vi "多影像平均_二值化_抓邊.vi"() -> ()   [LabVIEW 2015]
uses:
  <vilib>/vision/Measure.llb/Edge Options.ctl
  <vilib>/vision/Measure.llb/Edge Polarity.ctl
  <vilib>/userdefined/High Color/IMAQdx.ctl
  <vilib>/Utility/miscctls.llb/LVPositionTypeDef.ctl
  <vilib>/vision/NI_Vision_Development_Module.lvlib
  <vilib>/vision/driver/NI_Vision_Acquisition_Software.lvlib
  <resource>/objmgr/imaqdx.rc
panel:
  in  "Rectangle 2":T1={"Left"=208, "Top"=416, "Right"=273, "Bottom"=496, "Rotation"=0.0} {"Rotation" format="%.2f"; "Left" scale=0.0..1024.0; "Right" scale=0.0..1024.0}
  in  "載入影像":bool
  in  "拍攝影像":bool
  in  "影像數量":i32=4
  out "二值化影像陣列":T2[](array[plugin-control])
  out "全部影像Histograph":T3(graph)
  out "Image binary":T2(plugin-control)
  out "平均影像Histograph":T4(graph)
  out "Standard Deviation":sgl format="%#.2f"
  out "Mean":sgl format="%#.2f"
  out "影像陣列":T2[](array[plugin-control])
  in  "stop":bool
  in  "Horizontal Progress Bar":u8(slide) scale=0.0..255.0
  out "Image mean":T2(plugin-control)
  out "取像編號":i32
  out "取像視窗":T2(plugin-control)
  in  "Session In":T5="cam1"
  out "degrees":sgl
  in  "單點":bool
  in  "Edge Options":T6={"Edge Polarity"=0, "Kernel Size"=3, "Width"=3, "Minimum Edge Strength"=10.0, "Interpolation Type"=enum."Bilinear Fixed", "Data Processing Method"=enum."Average"} {"Edge Polarity" items=["All Edges", "Rising Edges", "Falling Edges"]; "Minimum Edge Strength" format="%.2f"; "Width" step=2; "Kernel Size" step=2}
  out "Gradient Information":dbl[][](graph)
  out "Line Segment":T8 {"Point 2"."Y" format="%.2f"; "Point 2"."X" format="%.2f"; "Point 1"."Y" format="%.2f"; "Point 1"."X" format="%.2f"}
  out "error out":errorcluster
  in  "Direction":T9(ring)
  in  "Process":u16(ring) items=["Get First Edge", "Get First + Last Edge", "Get All Edges", "Get Best Edge"]
  out "Line Profile":T10(graph)
  in  "Gap":i32=10 min=1 max=300
  out "Image":T2(plugin-control)
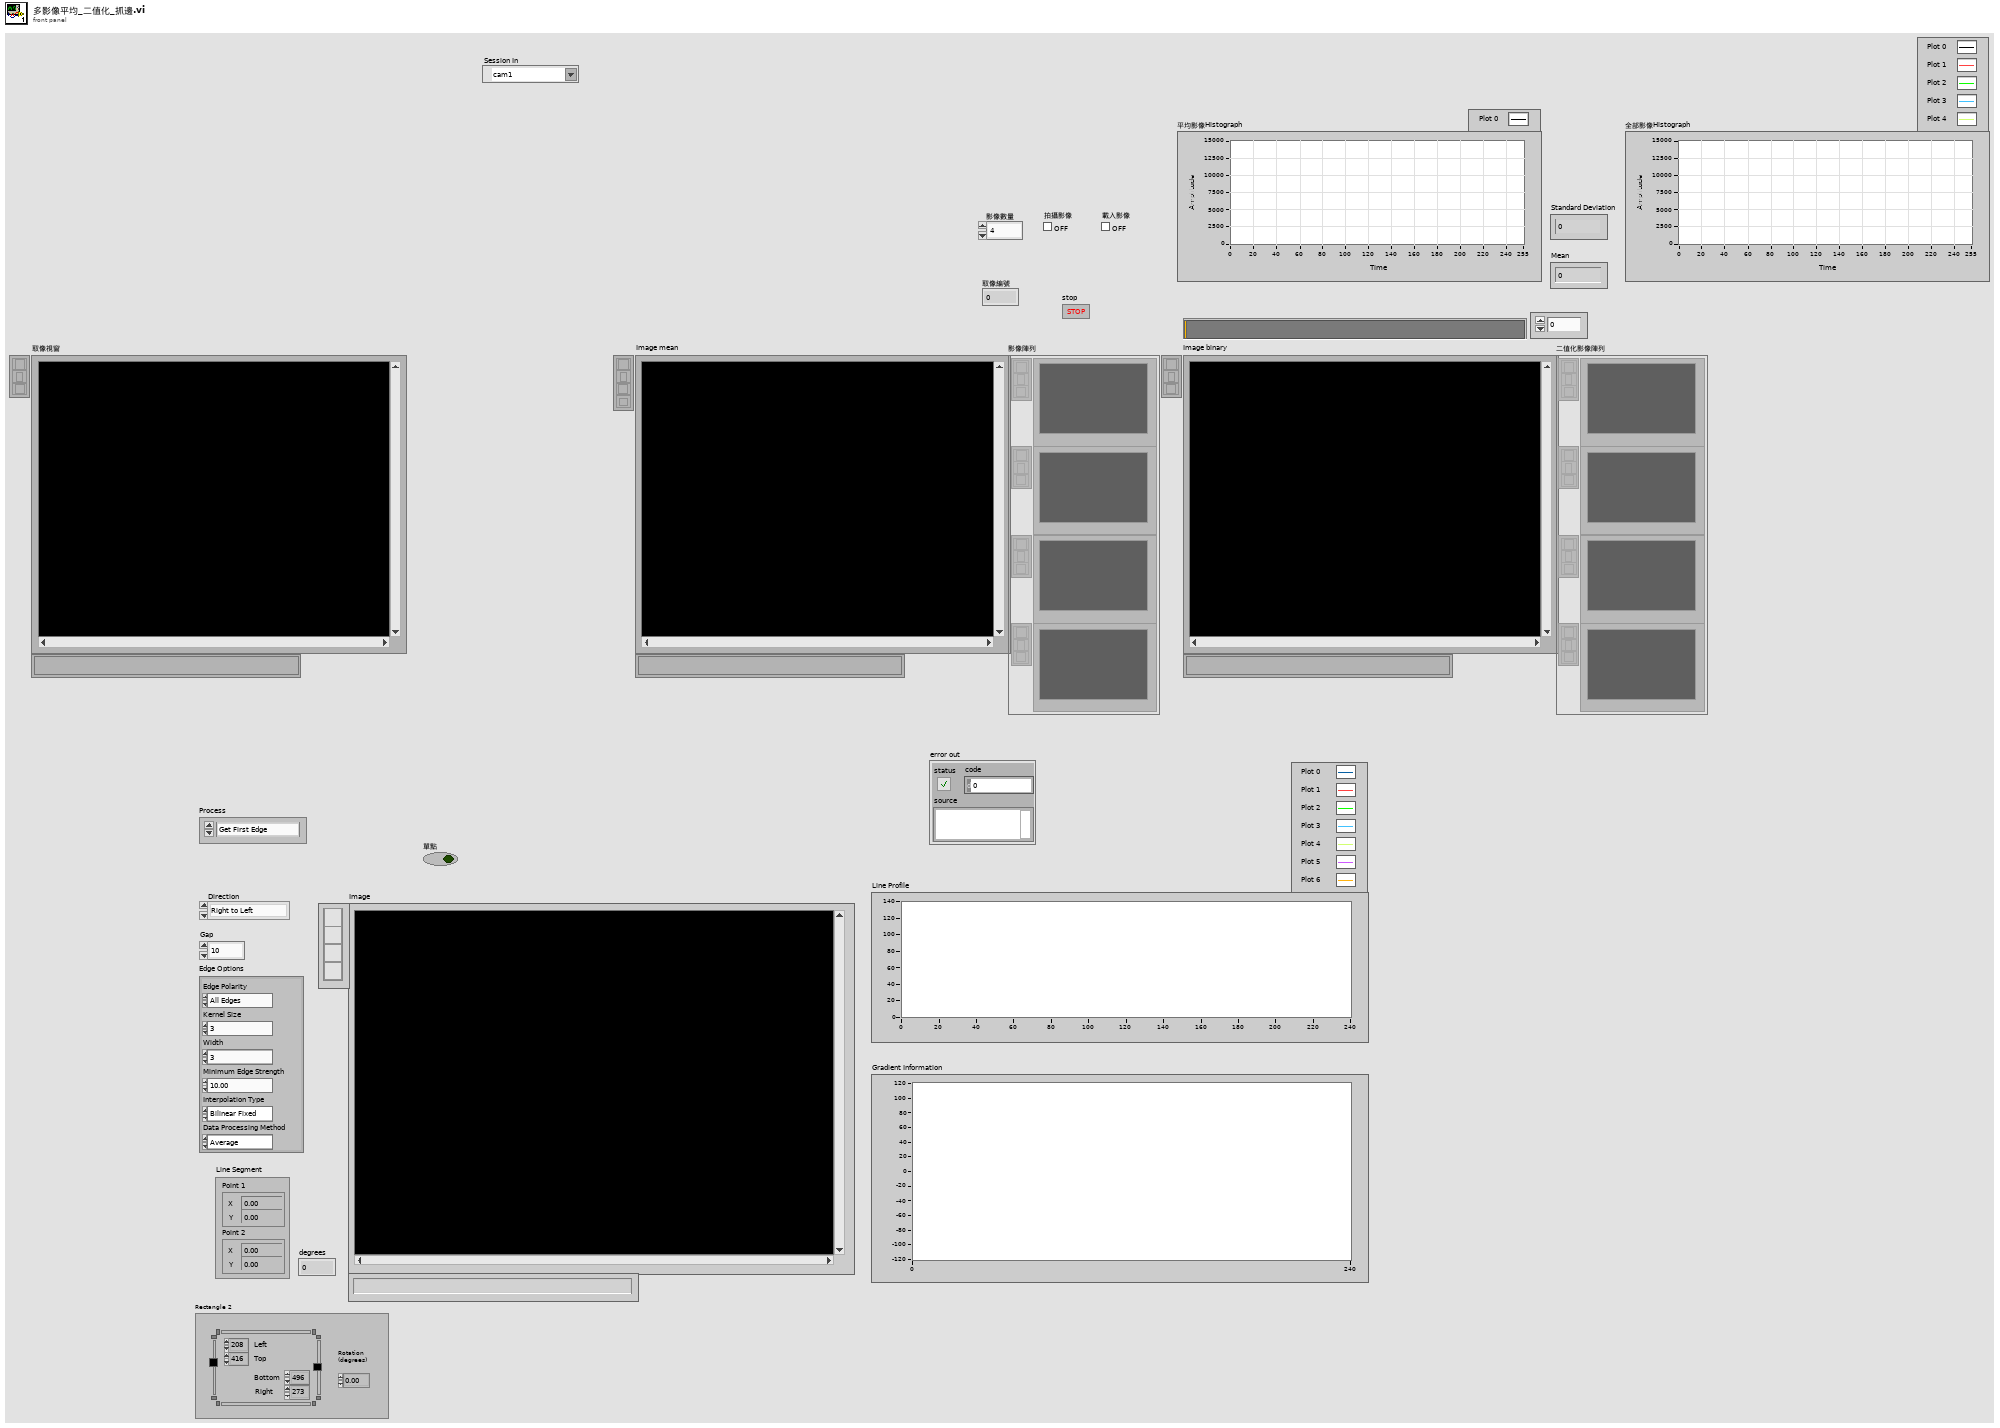
[diagram p1: front panel]
types:
  T1 = typedef "IMAQ Rectangle" = cluster{"Left":i32, "Top":i32, "Right":i32, "Bottom":i32, "Rotation":dbl}
  T2 = typedef "IMAQ Image.ctl" = refnum<image>
  T3 = cluster{"Starting Value":sgl, "Incremental Value":sgl, "Histogram":u32[]}[]
  T4 = cluster{"Starting Value":sgl, "Incremental Value":sgl, "Histogram":u32[]}
  T5 = typedef "IMAQdx.ctl" = refnum<k21>
  T6 = typedef "Edge Options.ctl" = cluster{"Edge Polarity":T7, "Kernel Size":u32, "Width":u32, "Minimum Edge Strength":sgl, "Interpolation Type":enum32{"Zero Order", "Bilinear", "Quadratic", "Cubic", "Bilinear Fixed"}, "Data Processing Method":enum32{"Average", "Median"}}
  T7 = typedef "Edge Polarity.ctl" = u32
  T8 = cluster{"Point 1":cluster{"X":sgl, "Y":sgl}, "Point 2":cluster{"X":sgl, "Y":sgl}}
  T9 = enum16{"Right to Left", "Left  to Right", "Up to Down", "Down to Up"}
  T10 = cluster{"x0":sgl, "dx":sgl, "Pixels Line":sgl[]}[]
  T11 = typedef "LVPositionTypeDef.ctl" = cluster{"Left":i32, "Top":i32}
  T12 = typedef "Image Type" = u32
  T13 = cluster{"Global Rectangle":i32[], "Contours":cluster{"Contour Type":u32, "ROI Type":u32, "Points":i32[]}[]}
  T14 = typedef "IMAQ Line" = cluster{"Start X":i32, "Start Y":i32, "End X":i32, "End Y":i32}
  T15 = cluster{"Point 1":cluster{"x":dbl, "y":dbl}, "Point 2":cluster{"x":dbl, "y":dbl}}
  T16 = typedef "ROI Descriptor" = cluster{"Global Rectangle":i32[], "Contours":cluster{"ID":enum32{"External", "Internal"}, "Type":u32, "Coordinates":i32[]}[]}
  T17 = typedef "IMAQ Point" = cluster{"X":sgl, "Y":sgl}
  T18 = typedef "Edge New.ctl" = cluster{"Location (Pixel)":cluster{"X":sgl, "Y":sgl}, "Location (Real-World)":cluster{"X":sgl, "Y":sgl}, "Distance (Pixel)":dbl, "Distance (Real-World)":dbl, "Strength":dbl, "Noise":dbl, "Rising?":bool}
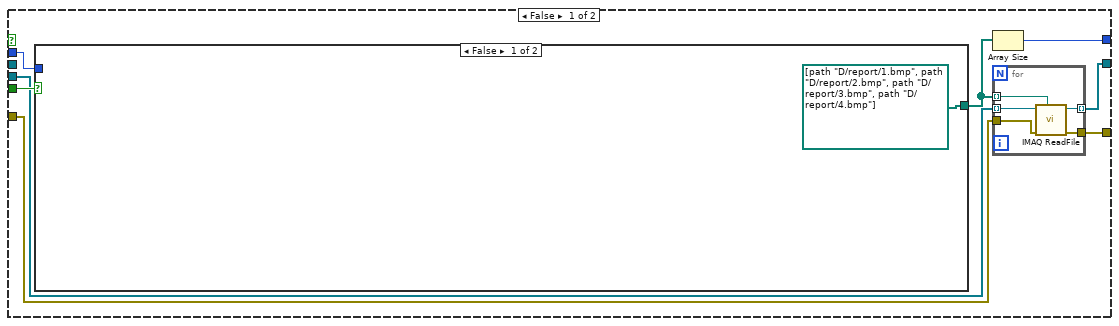
[diagram p2: hidden frame]
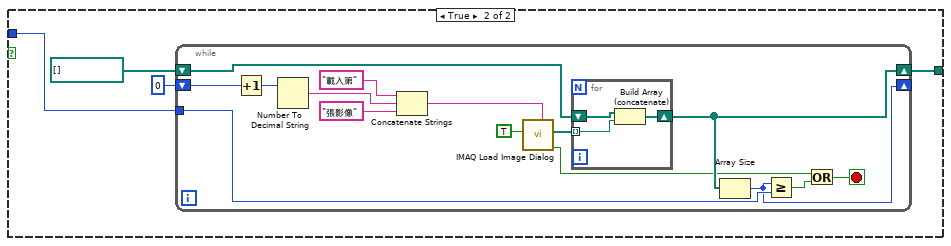
[diagram p3: hidden frame]
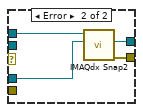
[diagram p4: hidden frame]
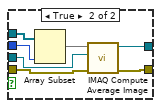
[diagram p5: hidden frame]
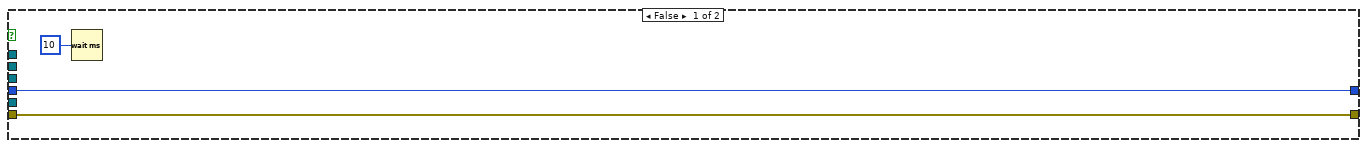
[diagram p6: hidden frame]
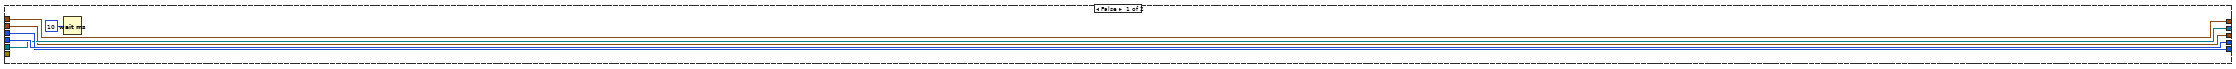
[diagram p8: hidden frame]
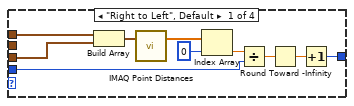
[diagram p9: hidden frame]
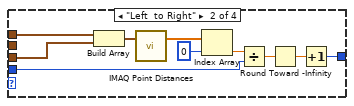
[diagram p10: hidden frame]
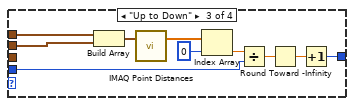
[diagram p11: hidden frame]
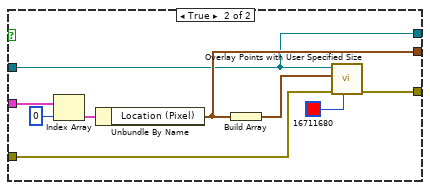
[diagram p14: hidden frame]
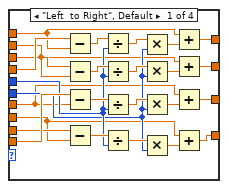
[diagram p15: hidden frame]
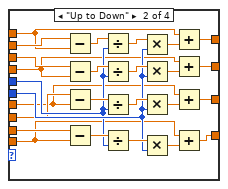
[diagram p16: hidden frame]
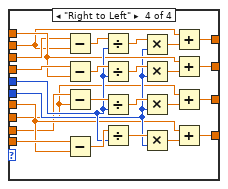
[diagram p17: hidden frame]
diagram:
  w40 = T12 0 items=["Grayscale (U8)", "Grayscale (I16)", "Grayscale (SGL)", "Complex (CSG)", "RGB (U32)", "HSL (U32)", "RGB (U64)", "Grayscale (U16)"] ("Image Type")
  w42 = i32[] [2] items=["No  event", "Click event", "Draw event", "Move event", "Size event", "Scroll event", "Activate event", "Close event", "Double click event"] ("Events list (all)")
  n1 = property on="Image" class="ImageControl"("ROI"=T13 {"Global Rectangle"=[450, 180, 600, 400], "Contours"=[{"Contour Type"=0, "ROI Type"=3, "Points"=[450, 180, 600, 400]}]}) -> ()  [unwired: 2 in, 2 out]
  n2 = property on="Pane" class="Pane"("Origin"=T11 {"Left"=-5267, "Top"=-1496} ("Position")) -> (error out=w5:errorcluster)  [unwired: 2 in, 1 out]
  n3 = flat-sequence {
    tunnel: [w68] -> w38
    tunnel: [w67] -> w37
    tunnel: [w65] -> w36
    tunnel: "影像數量" -> [w61]
    tunnel: [w63] -> w35
    tunnel: "拍攝影像" -> [w63]
    tunnel: [w62] -> w34
    tunnel: "載入影像" -> [w62]
    tunnel: [w61] -> w33
    tunnel: [w60] -> w32
    tunnel: [w57] -> w31
    tunnel: [w55] -> w30
    tunnel: [w53] -> w29
    tunnel: [w46] -> w28
    tunnel: w5 -> [w45]
    tunnel: w38 -> [w103]
    tunnel: w37 -> [w104]
    tunnel: [w102] -> w27
    tunnel: w36 -> [w101]
    tunnel: [w101] -> w26
    tunnel: w35 -> [w100]
    tunnel: w34 -> [w99]
    tunnel: w33 -> [w98]
    tunnel: [w97] -> w25
    tunnel: [w96] -> w24
    tunnel: w32 -> [w95]
    tunnel: [w95] -> w23
    tunnel: [w94] -> w22
    tunnel: w31 -> [w94]
    tunnel: w30 -> [w93]
    tunnel: [w93] -> w21
    tunnel: [w92] -> w20
    tunnel: w29 -> [w92]
    tunnel: w28 -> [w91]
    tunnel: w27 -> [w177]
    tunnel: w26 -> [w182]
    tunnel: w25 -> [w181]
    tunnel: w24 -> [w174]
    tunnel: w23 -> [w180]
    tunnel: [w180] -> w19
    tunnel: [w171] -> w18
    tunnel: [w177] -> w17
    tunnel: [w176] -> w16
    tunnel: [w179] -> w15
    tunnel: w22 -> [w179]
    tunnel: w21 -> [w175]
    tunnel: [w175] -> w14
    tunnel: [w178] -> w13
    tunnel: w20 -> [w178]
    tunnel: w19 -> [w202]
    tunnel: w18 -> [w197]
    tunnel: w17 -> [w203]
    tunnel: w16 -> [w195]
    tunnel: w15 -> [w201]
    tunnel: w14 -> [w196]
    tunnel: w13 -> [w198]
    tunnel: [w195] -> w9
    tunnel: [w194] -> w4
    frame #0 {
      w59 = T12 0 items=["Grayscale (U8)", "Grayscale (I16)", "Grayscale (SGL)", "Complex (CSG)", "RGB (U32)", "HSL (U32)", "RGB (U64)", "Grayscale (U16)"] ("Image Type")
      w52 = 20
      w64 = T12 0 items=["Grayscale (U8)", "Grayscale (I16)", "Grayscale (SGL)", "Complex (CSG)", "RGB (U32)", "HSL (U32)", "RGB (U64)", "Grayscale (U16)"] ("Image Type")
      n4 = call <vilib>:"IMAQdx Open Camera.vi"("error in"=w45, "Session In"="Session In") -> ("error out"=w54:errorcluster, "Session Out"=w68:T5)  [unwired: 8 in]
      n5 = for {
        N: w52 -> [_]
        tunnel: [w90] -> w67 mode=indexing
        tunnel: w54 -> [w89]
        tunnel: [w88] -> w51
        i -> [w87]
        n6 = Number To Decimal String(number=w87) -> (decimal integer string=w85:string)  [unwired: 1 in]
        n7 = Concatenate Strings("Image", w85) -> (w84:string)
        n8 = call "IMAQ Create"("Image Name"=w84, "error in (no error)"=w89) -> ("New Image"=w90:T2, "error out"=w88:errorcluster)  [unwired: 3 in]
      }
      n9 = for {
        N: w52 -> [_]
        tunnel: [w76] -> w53 mode=indexing
        tunnel: w51 -> [w75]
        tunnel: [w70] -> _
        tunnel: [w70] -> w50 mode=indexing
        i -> [w74]
        n10 = Number To Decimal String(number=w74) -> (decimal integer string=w72:string)  [unwired: 1 in]
        n11 = Concatenate Strings("Histogram Mask", w72) -> (w71:string)
        n12 = call "IMAQ Create"("Image Name"=w71, "error in (no error)"=w75) -> ("New Image"=w76:T2, "error out"=w70:errorcluster)  [unwired: 3 in]
      }
      n13 = for {
        N: w52 -> [_]
        tunnel: [w83] -> w60 mode=indexing
        tunnel: w50 -> [w82] mode=indexing
        tunnel: [w81] -> w47
        i -> [w80]
        n14 = Number To Decimal String(number=w80) -> (decimal integer string=w78:string)  [unwired: 1 in]
        n15 = Concatenate Strings("Threshole", w78) -> (w77:string)
        n16 = call "IMAQ Create"("Image Name"=w77, "error in (no error)"=w82) -> ("New Image"=w83:T2, "error out"=w81:errorcluster)  [unwired: 3 in]
      }
      n17 = call "IMAQ Create"("Image Name"="imageMeans", "Image Type"=w64, "error in (no error)"=w47) -> ("New Image"=w65:T2, "error out"=w49:errorcluster)  [unwired: 2 in]
      n18 = call "IMAQ Create"("Image Name"="Histogram Mask", "error in (no error)"=w49) -> ("New Image"=w55:T2, "error out"=w48:errorcluster)  [unwired: 3 in]
      n19 = call "IMAQ Create"("Image Name"="imageBinary", "Image Type"=w59, "error in (no error)"=w48) -> ("New Image"=w57:T2, "error out"=w46:errorcluster)  [unwired: 2 in]
    }
    frame #1 {
      n20 = case shown="True" w100 {
        tunnel: w104 -> [w109 w148]
        tunnel: w103 -> [_ w147]
        tunnel: w91 -> [w108 w145]
        tunnel: [w110 w144] -> w102
        tunnel: w99 -> [w112 _]
        tunnel: w98 -> [w111 w142]
        tunnel: [w107 w143] -> w97
        tunnel: [w105 w142] -> w96
        frame False {
          n21 = case shown="False" w112 {
            tunnel: [path[] [path "D:/report/1.bmp", path "D:/report/2.bmp", path "D:/report/3.bmp", path "D:/report/4.bmp"] w117] -> w106
            tunnel: w111 -> [_ w116]
            frame False {
            }
            frame True {
              n22 = while {
                tunnel: w116 -> [w129]
                shift-right: [w132] -> w117
                shift-left: path[] [] -> [w128]
                shift-right: [w127] -> _
                shift-left: 0 -> [w126]
                stop <- w119 stop-if-true
                n23 = Increment(x=w126) -> (x+1=w125:i32)
                n24 = Number To Decimal String(number=w125) -> (decimal integer string=w122:string)  [unwired: 1 in]
                n25 = Concatenate Strings("載入第", w122, "張影像") -> (w121:string)
                n26 = call "IMAQ Load Image Dialog"("Button Label"=w121, "Multiple Files? (No)"=TRUE) -> ("Cancelled?"=w120:bool, "Paths"=w130:path[])  [unwired: 7 in, 1 out]
                n27 = for {
                  tunnel: w130 -> [w134] mode=indexing
                  shift-right: [w133] -> w132
                  shift-left: w128 -> [w135]
                  n28 = Build Array (concatenate)(w135, w134) -> (w133:path[])
                }
                n29 = Array Size(array=w132) -> (size(s)=w127:i32)
                n30 = Greater Or Equal?(x=w127, y=w129) -> (x >= y?=w118:bool)
                n31 = Or(x=w120, y=w118) -> (x .or. y?=w119:bool)
              }
            }
          }
          n32 = Array Size(array=w106) -> (size(s)=w105:i32)
          n33 = for {
            tunnel: w106 -> [w140] mode=indexing
            tunnel: [w139] -> w110 mode=indexing
            tunnel: w109 -> [w138] mode=indexing
            tunnel: w108 -> [w137]
            tunnel: [w136] -> w107
            n34 = call "IMAQ ReadFile"("File Path"=w140, "error in (no error)"=w137, "Image"=w138) -> ("error out"=w136:errorcluster, "Image Out"=w139:T2)  [unwired: 4 in, 3 out]
          }
        }
        frame True {
          n35 = for {
            N: w142 -> [_]
            tunnel: w148 -> [w151] mode=indexing
            tunnel: w147 -> [w149]
            tunnel: dbl[] [0.01, 0.03, 0.05, 0.07] -> [w159] mode=indexing
            tunnel: w145 -> [w154]
            tunnel: [w158] -> w144 mode=indexing
            tunnel: [w156] -> w143
            i -> [w160]
            w157 = T12 0 items=["Grayscale (U8)", "Grayscale (I16)", "Grayscale (SGL)", "Complex (CSG)", "RGB (U32)", "HSL (U32)", "RGB (U64)", "Grayscale (U16)"] ("Image Type")
            n36 = property class="IMAQdx"(reference=w149, error in=w154, "ActiveAttribute"="CameraAttributes::Exposure::Value", "ValueDBL"=w159) -> (reference out=w150:T5, error out=w152:errorcluster)
            n37 = case shown="No Error" w152 {
              tunnel: [w165 w169] -> w156
              tunnel: [w164 w166] -> w155
              tunnel: w152 -> [w163 _]
              tunnel: w150 -> [w162 _]
              tunnel: w151 -> [w161 w168]
              tunnel: w149 -> [_ w167]
              frame No Error {
                n38 = call <vilib>:"IMAQdx Snap2.vi"("error in"=w163, "Image In"=w161, "Session In"=w162) -> ("error out"=w165:errorcluster, "Image Out"=w164:T2)  [unwired: 6 in, 1 out]
              }
              frame Error {
                n39 = call <vilib>:"IMAQdx Snap2.vi"("Image In"=w168, "Session In"=w167) -> ("error out"=w169:errorcluster, "Image Out"=w166:T2)  [unwired: 7 in, 1 out]
              }
            }
            "取像視窗" <- w155
            n40 = call "IMAQ Cast Image"("Image Type"=w157, "Image Src"=w155) -> ("Image Dst Out"=w158:T2)  [unwired: 8 in, 1 out]
            "取像編號" <- w160
          }
          n41 = property on="Pane" class="Pane"("Origin"=T11 {"Left"=-6573, "Top"=-1496} ("Position")) -> ()  [unwired: 2 in, 2 out]
        }
      }
    }
    frame #2 {
      n42 = Not Equal?(x=w174, y=1) -> (x != y?=w172:bool)
      n43 = case shown="False" w172 {
        tunnel: w182 -> [_ w193]
        tunnel: w181 -> [w186 w192]
        tunnel: w174 -> [_ w191]
        tunnel: [w186 w189] -> w171
        tunnel: w177 -> [w184 w188]
        tunnel: [w183 w187] -> w176
        frame False {
          n44 = Index Array(array=w184, index=0) -> (element=w183:T2)
        }
        frame True {
          n45 = Array Subset(array=w188, length=w191) -> (w190:T2[])  [unwired: 1 in]
          n46 = call "IMAQ Compute Average Image"("error in (no error)"=w192, "Image Dst"=w193, "Images"=w190) -> ("error out"=w189:errorcluster, "Image Dst Out"=w187:T2)  [unwired: 7 in]
        }
      }
      "Image mean" <- w176
      n47 = property on="Pane" class="Pane"("Origin"=T11 {"Left"=-5267, "Top"=-1496} ("Position")) -> ()  [unwired: 2 in, 2 out]
    }
    frame #3 {
      w199 = i32[] [2] items=["No  event", "Click event", "Draw event", "Move event", "Size event", "Scroll event", "Activate event", "Close event", "Double click event"] ("Events list (all)")
      n48 = property on="Image mean" class="ImageControl"("ROI"=T13 {"Global Rectangle"=[0, 0, 1292, 964], "Contours"=[{"Contour Type"=0, "ROI Type"=3, "Points"=[0, 0, 1292, 964]}]}) -> ()  [unwired: 2 in, 2 out]
      n49 = while {
        tunnel: w203 -> [w223]
        tunnel: w202 -> [w222]
        tunnel: w195 -> [w220]
        tunnel: w196 -> [w221]
        tunnel: w201 -> [w219]
        tunnel: w199 -> [w217]
        shift-right: [w214] -> _
        shift-left: _ -> [w212]
        tunnel: w198 -> [w207]
        tunnel: w197 -> [w206]
        tunnel: [w204] -> w194
        i -> [w215]
        stop <- "stop" stop-if-true
        n50 = invoke on="Image mean" class="ImageControl" method="Get Last Event"("Which Events"=w217) -> ("Type"=w216:i32)  [unwired: 7 in, 7 out]
        n51 = property on="平均影像Histograph" class="WFGraph (strict)"() -> ("YScale.Maximum"=w205:dbl)  [unwired: 2 in, 2 out]
        n52 = property on="全部影像Histograph" class="WFGraph (strict)"("YScale.Maximum"=w205) -> ()  [unwired: 2 in, 2 out]
        n53 = Not Equal?(x="Horizontal Progress Bar", y=w212) -> (x != y?=w209:bool)
        n54 = Not Equal To 0?(x=w216) -> (x != 0?=w210:bool)
        n55 = Equal To 0?(x=w215) -> (x = 0?=w211:bool)
        n56 = Compound Arithmetic op=OR(w211, w210, w209) -> (w208:bool)
        n57 = case shown="True" w208 {
          tunnel: w223 -> [_ w232]
          tunnel: w222 -> [_ w260]
          tunnel: w221 -> [_ w229]
          tunnel: w220 -> [_ w230]
          tunnel: w219 -> [_ w247]
          tunnel: "Horizontal Progress Bar" -> [w225 w245]
          tunnel: [w225 w245] -> w214
          tunnel: w207 -> [_ w243]
          tunnel: w206 -> [w224 w234]
          tunnel: [w224 w227] -> w204
          frame False {
            n58 = Wait (ms)(milliseconds to wait=u32 10) -> ()  [unwired: 1 out]
          }
          frame True {
            n59 = property on="Image mean" class="ImageControl"() -> ("ROI"=w242:T13)  [unwired: 2 in, 2 out]
            n60 = property on="Image binary" class="ImageControl"("Zoom to Fit Mode"=TRUE) -> ()  [unwired: 2 in, 2 out]
            n61 = call "IMAQ Convert ROI to Rectangle"("error in (no error)"=w234, "ROI Descriptor"=w242) -> ("error out"=w235:errorcluster, "Rectangle"=w252:T1)  [unwired: 7 in]
            n62 = Unbundle By Name(w252) -> ("Left"=w248:i32, "Top"=w249:i32, "Right"=w250:i32, "Bottom"=w251:i32)
            n63 = Build Array(w248, w249, w250, w251) -> (w241:i32[])
            n64 = for {
              tunnel: w232 -> [w263] mode=indexing
              tunnel: w260 -> [w277] mode=indexing
              tunnel: [w276] -> w259 mode=indexing
              tunnel: [w264] -> w255 mode=indexing
              tunnel: w245 -> [w273]
              tunnel: w243 -> [w270] mode=indexing
              tunnel: w242 -> [w272]
              tunnel: w241 -> [w271]
              tunnel: [w267] -> w236
              tunnel: w235 -> [w266]
              tunnel: [w265] -> w231 mode=indexing
              n65 = call "IMAQ ROIToMask"("error in (no error)"=w266, "ROI Descriptor"=w272, "Image"=w270, "Image Model"=w263) -> ("error out"=w269:errorcluster, "Image Out"=w262:T2)  [unwired: 2 in, 1 out]
              n66 = call "IMAQ Extract 2"("Optional Rectangle"=w271, "error in (no error)"=w269, "Image Dst"=w270, "Image Src"=w263) -> ("error out"=w268:errorcluster, "Image Dst Out"=w265:T2)  [unwired: 6 in]
              n67 = Bundle By Name(cluster=cluster{"Lower value":sgl, "Upper value":sgl} {"Lower value"=128.0, "Upper value"=255.0} ("Range"), "Lower value"=w273) -> (w274:cluster{"Lower value":sgl, "Upper value":sgl})
              n68 = call "IMAQ Histograph"("error in (no error)"=w268, "Image"=w262) -> ("error out"=w261:errorcluster, "Histogram Graph"=w264:T4)  [unwired: 6 in, 2 out]
              n69 = call "IMAQ Threshold"("error in (no error)"=w261, "Range"=w274, "Image Dst"=w277, "Image Src"=w265) -> ("error out"=w267:errorcluster, "Image Dst Out"=w276:T2)  [unwired: 6 in]
            }
            "二值化影像陣列" <- w259
            "影像陣列" <- w231
            n70 = call "IMAQ ROIToMask"("error in (no error)"=w236, "ROI Descriptor"=w242, "Image"=w229, "Image Model"=w230) -> ("error out"=w239:errorcluster, "Image Out"=w228:T2)  [unwired: 2 in, 1 out]
            n71 = call "IMAQ Extract 2"("Optional Rectangle"=w241, "error in (no error)"=w239, "Image Dst"=w229, "Image Src"=w230) -> ("error out"=w238:errorcluster, "Image Dst Out"=w240:T2)  [unwired: 6 in]
            n72 = call "IMAQ Histograph"("error in (no error)"=w238, "Image"=w228) -> ("error out"=w237:errorcluster, "Standard  Deviation"=→"Standard Deviation":sgl, "Mean Value"=→"Mean":sgl, "Histogram Graph"=w253:T4)  [unwired: 6 in]
            "平均影像Histograph" <- w253
            n73 = Bundle By Name(cluster=cluster{"Lower value":sgl, "Upper value":sgl} {"Lower value"=128.0, "Upper value"=255.0} ("Range"), "Lower value"=w245) -> (w258:cluster{"Lower value":sgl, "Upper value":sgl})
            n74 = Build Array (concatenate)(w253, w255) -> (→"全部影像Histograph":T3)
            n75 = call "IMAQ Threshold"("error in (no error)"=w237, "Range"=w258, "Image Dst"=w247, "Image Src"=w240) -> ("error out"=w227:errorcluster, "Image Dst Out"=→"Image binary":T2)  [unwired: 6 in]
          }
        }
      }
    }
  }
  n76 = property on="Pane" class="Pane"(error in=w4, "Origin"=T11 {"Left"=-5844, "Top"=-513} ("Position")) -> (error out=w3:errorcluster)  [unwired: 1 in, 1 out]
  n77 = call "IMAQ Create"("Image Name"="Edge Detection Source", "error in (no error)"=w3) -> ("New Image"=w7:T2, "error out"=w6:errorcluster)  [unwired: 3 in]
  n78 = call "IMAQ Copy"("Image Dst"=w7, "Image Src"=w9) -> ("Image Dst Out"=w8:T2)  [unwired: 4 in, 1 out]
  n79 = call "IMAQ Cast Image"("Image Type"=w40, "error in (no error)"=w6, "Image Src"=w8) -> ("error out"=w39:errorcluster, "Image Dst Out"=w41:T2)  [unwired: 7 in]
  n80 = while {
    tunnel: w39 -> [w299]
    tunnel: w41 -> [w300]
    tunnel: w42 -> [w282]
    shift-right: [w297] -> _
    shift-left: _ -> [w296]
    shift-right: [w289] -> _
    shift-left: _ -> [w290]
    shift-right: [w284] -> _
    shift-left: _ -> [w285]
    shift-right: [w281] -> _
    shift-left: _ -> [w280]
    stop <- FALSE stop-if-true
    n81 = invoke on="Image" class="ImageControl" method="Get Last Event"("Which Events"=w282) -> ("Type"=w298:i32)  [unwired: 7 in, 7 out]
    n82 = Not Equal?(x=w285, y="Edge Options") -> (x != y?=w283:bool)
    n83 = Not Equal?(x=w280, y="Rectangle 2") -> (x != y?=w278:bool)
    n84 = Not Equal?(x=w296, y="Direction") -> (x != y?=w295:bool)
    n85 = Not Equal?(x=w290, y="Gap") -> (x != y?=w288:bool)
    n86 = Not Equal To 0?(x=w298) -> (x != 0?=w294:bool)
    n87 = case shown="True" w278 {
      tunnel: "Rectangle 2" -> [_ w303]
      frame False {
      }
      frame True {
        n88 = call "IMAQ Convert Rectangle to ROI"("Rectangle"=w303) -> ("ROI Descriptor"=w302:T16)  [unwired: 8 in, 1 out]
        n89 = property on="Image" class="ImageControl"("ROI"=w302) -> ()  [unwired: 2 in, 2 out]
      }
    }
    n90 = Compound Arithmetic op=OR(w295, w294, w288, w283, w278) -> (w293:bool)
    n91 = case shown="True" w293 {
      tunnel: w300 -> [w306 w362]
      tunnel: w299 -> [_ w361]
      tunnel: "Direction" -> [w308 w353]
      tunnel: [w308 w353] -> w297
      tunnel: "Gap" -> [w307 w352]
      tunnel: [w307 w352] -> w289
      tunnel: [w306 w323] -> w287
      tunnel: "Edge Options" -> [w305 w332]
      tunnel: [w305 w332] -> w284
      tunnel: [w304 w310] -> w281
      tunnel: w280 -> [w304 _]
      frame False {
        n92 = Wait (ms)(milliseconds to wait=u32 10) -> ()  [unwired: 1 out]
      }
      frame True {
        n93 = call "IMAQ Clear Overlay"("error in (no error)"=w361, "Image"=w362) -> ("error out"=w360:errorcluster, "Image Out"=w335:T2)  [unwired: 8 in]
        n94 = property on="Image" class="ImageControl"() -> ("ROI"=w363:T13)  [unwired: 2 in, 2 out]
        n95 = call "IMAQ Convert ROI to Rectangle"("error in (no error)"=w360, "ROI Descriptor"=w363) -> ("error out"=w334:errorcluster, "Rectangle"=w310:T1)  [unwired: 7 in]
        n96 = local write "Rectangle 2"(w310) -> ()
        n97 = call "IMAQ Convert Rectangle to ROI (Polygon)"("Rectangle"=w310) -> ("Rectangle Points"=w349:T17[])  [unwired: 7 in, 2 out]
        n98 = Index Array(array=w349, index #1=0 ("index"), index #2=1 ("index"), index #3=2 ("index"), index #4=3 ("index")) -> (element #1=w351:T17, element #2=w350:T17, element #3=w341:T17, element #4=w342:T17)
        n99 = case shown="\"Down to Up\"" w353 {
          tunnel: w352 -> [w371 w381 w391 w401]
          tunnel: [w370 w380 w390 w400] -> w348
          tunnel: w351 -> [w367 w377 w389 w397]
          tunnel: w342 -> [w366 w376 _ _]
          tunnel: w350 -> [_ _ w385 w396]
          frame "Right to Left", Default {
            n100 = Build Array(w367, w366) -> (w369:T17[])
            n101 = call "IMAQ Point Distances"("Points"=w369) -> ("Distances"=w368:sgl[])  [unwired: 4 in, 1 out]
            n102 = Index Array(array=w368, index=0) -> (element=w364:sgl)
            n103 = Divide(x=w364, y=w371) -> (x/y=w372:sgl)
            n104 = Round Toward -Infinity(1:w372) -> (0:w373:sgl)
            n105 = Increment(x=w373) -> (x+1=w370:i32)
          }
          frame "Left  to Right" {
            n106 = Build Array(w377, w376) -> (w379:T17[])
            n107 = call "IMAQ Point Distances"("Points"=w379) -> ("Distances"=w378:sgl[])  [unwired: 4 in, 1 out]
            n108 = Index Array(array=w378, index=0) -> (element=w374:sgl)
            n109 = Divide(x=w374, y=w381) -> (x/y=w382:sgl)
            n110 = Round Toward -Infinity(1:w382) -> (0:w383:sgl)
            n111 = Increment(x=w383) -> (x+1=w380:i32)
          }
          frame "Up to Down" {
            n112 = Build Array(w389, w385) -> (w388:T17[])
            n113 = call "IMAQ Point Distances"("Points"=w388) -> ("Distances"=w387:sgl[])  [unwired: 4 in, 1 out]
            n114 = Index Array(array=w387, index=0) -> (element=w386:sgl)
            n115 = Divide(x=w386, y=w391) -> (x/y=w392:sgl)
            n116 = Round Toward -Infinity(1:w392) -> (0:w393:sgl)
            n117 = Increment(x=w393) -> (x+1=w390:i32)
          }
          frame "Down to Up" {
            n118 = Build Array(w397, w396) -> (w399:T17[])
            n119 = call "IMAQ Point Distances"("Points"=w399) -> ("Distances"=w398:sgl[])  [unwired: 4 in, 1 out]
            n120 = Index Array(array=w398, index=0) -> (element=w395:sgl)
            n121 = Divide(x=w395, y=w401) -> (x/y=w402:sgl)
            n122 = Round Toward -Infinity(1:w402) -> (0:w403:sgl)
            n123 = Increment(x=w403) -> (x+1=w400:i32)
          }
        }
        n124 = Unbundle By Name(w351) -> ("X"=w346:sgl, "Y"=w345:sgl)
        n125 = Unbundle By Name(w350) -> ("X"=w339:sgl, "Y"=w337:sgl)
        n126 = Unbundle By Name(w341) -> ("X"=w340:sgl, "Y"=w338:sgl)
        n127 = Unbundle By Name(w342) -> ("X"=w347:sgl, "Y"=w336:sgl)
        n128 = for {
          N: w348 -> [w436]
          tunnel: w353 -> [w428]
          tunnel: w347 -> [w464]
          tunnel: w346 -> [w463]
          tunnel: w336 -> [w462]
          tunnel: w345 -> [w461]
          tunnel: w340 -> [w460]
          tunnel: w339 -> [w459]
          tunnel: w338 -> [w458]
          tunnel: w337 -> [w457]
          tunnel: [w448] -> w328
          tunnel: w335 -> [w431]
          tunnel: w334 -> [w420]
          tunnel: [w446] -> w327
          tunnel: "Process" -> [w449]
          tunnel: w332 -> [w445]
          tunnel: [w443] -> w331 mode=indexing
          tunnel: [w442] -> w330 mode=indexing
          tunnel: [w441] -> w329 mode=indexing
          i -> [w437]
          w435 = 1
          w421 = u32 16860 ("Color")
          w426 = cluster{"X":i32, "Y":i32} {"X"=0, "Y"=0} ("Start Point")
          n129 = Equal?(x=w437, y=w435) -> (x = y?=w433:bool)
          n130 = Subtract(x=w436, y=w435) -> (x-y=w434:i32)
          n131 = case shown="\"Down to Up\"" w428 {
            tunnel: [w509 w528 w554 w579] -> w456
            tunnel: [w504 w527 w553 w580] -> w425
            tunnel: [w507 w525 w551 w577] -> w455
            tunnel: [w503 w526 w552 w578] -> w427
            tunnel: w464 -> [w522 w533 w559 w589]
            tunnel: w463 -> [w500 w535 w558 w588]
            tunnel: w436 -> [w513 w537 w564 w590]
            tunnel: w437 -> [w512 w538 w555 w587]
            tunnel: w462 -> [w519 w529 w561 w584]
            tunnel: w461 -> [w502 w531 w560 w583]
            tunnel: w460 -> [w516 w534 w557 w586]
            tunnel: w459 -> [w501 w536 w556 w585]
            tunnel: w458 -> [w511 w530 w562 w582]
            tunnel: w457 -> [w499 w532 w563 w581]
            frame "Left  to Right", Default {
              n132 = Subtract(x=w522, y=w500) -> (x-y=w523:sgl)
              n133 = Subtract(x=w516, y=w501) -> (x-y=w518:sgl)
              n134 = Subtract(x=w519, y=w502) -> (x-y=w521:sgl)
              n135 = Subtract(x=w511, y=w499) -> (x-y=w514:sgl)
              n136 = Divide(x=w523, y=w513) -> (x/y=w524:sgl)
              n137 = Divide(x=w518, y=w513) -> (x/y=w517:sgl)
              n138 = Divide(x=w521, y=w513) -> (x/y=w520:sgl)
              n139 = Divide(x=w514, y=w513) -> (x/y=w515:sgl)
              n140 = Multiply(x=w524, y=w512) -> (x*y=w510:sgl)
              n141 = Multiply(x=w517, y=w512) -> (x*y=w506:sgl)
              n142 = Multiply(x=w520, y=w512) -> (x*y=w508:sgl)
              n143 = Multiply(x=w515, y=w512) -> (x*y=w505:sgl)
              n144 = Add(x=w500, y=w510) -> (x+y=w509:sgl)
              n145 = Add(x=w501, y=w506) -> (x+y=w504:sgl)
              n146 = Add(x=w502, y=w508) -> (x+y=w507:sgl)
              n147 = Add(x=w499, y=w505) -> (x+y=w503:sgl)
            }
            frame "Up to Down" {
              n148 = Subtract(x=w536, y=w535) -> (x-y=w549:sgl)
              n149 = Subtract(x=w534, y=w533) -> (x-y=w546:sgl)
              n150 = Subtract(x=w532, y=w531) -> (x-y=w548:sgl)
              n151 = Subtract(x=w530, y=w529) -> (x-y=w543:sgl)
              n152 = Divide(x=w549, y=w537) -> (x/y=w550:sgl)
              n153 = Divide(x=w546, y=w537) -> (x/y=w545:sgl)
              n154 = Divide(x=w548, y=w537) -> (x/y=w547:sgl)
              n155 = Divide(x=w543, y=w537) -> (x/y=w544:sgl)
              n156 = Multiply(x=w550, y=w538) -> (x*y=w542:sgl)
              n157 = Multiply(x=w545, y=w538) -> (x*y=w540:sgl)
              n158 = Multiply(x=w547, y=w538) -> (x*y=w541:sgl)
              n159 = Multiply(x=w544, y=w538) -> (x*y=w539:sgl)
              n160 = Add(x=w535, y=w542) -> (x+y=w528:sgl)
              n161 = Add(x=w533, y=w540) -> (x+y=w527:sgl)
              n162 = Add(x=w531, y=w541) -> (x+y=w525:sgl)
              n163 = Add(x=w529, y=w539) -> (x+y=w526:sgl)
            }
            frame "Down to Up" {
              n164 = Subtract(x=w557, y=w559) -> (x-y=w572:sgl)
              n165 = Subtract(x=w556, y=w558) -> (x-y=w575:sgl)
              n166 = Subtract(x=w562, y=w561) -> (x-y=w569:sgl)
              n167 = Subtract(x=w563, y=w560) -> (x-y=w574:sgl)
              n168 = Divide(x=w572, y=w564) -> (x/y=w571:sgl)
              n169 = Divide(x=w575, y=w564) -> (x/y=w576:sgl)
              n170 = Divide(x=w569, y=w564) -> (x/y=w570:sgl)
              n171 = Divide(x=w574, y=w564) -> (x/y=w573:sgl)
              n172 = Multiply(x=w571, y=w555) -> (x*y=w566:sgl)
              n173 = Multiply(x=w576, y=w555) -> (x*y=w568:sgl)
              n174 = Multiply(x=w570, y=w555) -> (x*y=w565:sgl)
              n175 = Multiply(x=w573, y=w555) -> (x*y=w567:sgl)
              n176 = Add(x=w559, y=w566) -> (x+y=w554:sgl)
              n177 = Add(x=w558, y=w568) -> (x+y=w553:sgl)
              n178 = Add(x=w561, y=w565) -> (x+y=w551:sgl)
              n179 = Add(x=w560, y=w567) -> (x+y=w552:sgl)
            }
            frame "Right to Left" {
              n180 = Subtract(x=w586, y=w585) -> (x-y=w598:sgl)
              n181 = Subtract(x=w589, y=w588) -> (x-y=w601:sgl)
              n182 = Subtract(x=w582, y=w581) -> (x-y=w595:sgl)
              n183 = Subtract(x=w584, y=w583) -> (x-y=w600:sgl)
              n184 = Divide(x=w598, y=w590) -> (x/y=w597:sgl)
              n185 = Divide(x=w601, y=w590) -> (x/y=w602:sgl)
              n186 = Divide(x=w595, y=w590) -> (x/y=w596:sgl)
              n187 = Divide(x=w600, y=w590) -> (x/y=w599:sgl)
              n188 = Multiply(x=w597, y=w587) -> (x*y=w592:sgl)
              n189 = Multiply(x=w602, y=w587) -> (x*y=w594:sgl)
              n190 = Multiply(x=w596, y=w587) -> (x*y=w591:sgl)
              n191 = Multiply(x=w599, y=w587) -> (x*y=w593:sgl)
              n192 = Add(x=w585, y=w592) -> (x+y=w579:sgl)
              n193 = Add(x=w588, y=w594) -> (x+y=w580:sgl)
              n194 = Add(x=w581, y=w591) -> (x+y=w577:sgl)
              n195 = Add(x=w583, y=w593) -> (x+y=w578:sgl)
            }
          }
          n196 = Equal?(x=w437, y=w434) -> (x = y?=w432:bool)
          n197 = Or(x=w433, y=w432) -> (x .or. y?=w423:bool)
          n198 = Bundle By Name(cluster=w426, "X"=w425, "Y"=w427) -> (w424:cluster{"X":i32, "Y":i32})
          n199 = Bundle By Name(cluster=w426, "X"=w456, "Y"=w455) -> (w422:cluster{"X":i32, "Y":i32})
          n200 = Bundle By Name(cluster=T14 {"Start X"=0, "Start Y"=0, "End X"=0, "End Y"=0} ("Line"), "Start X"=w456, "Start Y"=w455, "End X"=w425, "End Y"=w427) -> (w444:T14)
          n201 = case shown="True" w423 {
            tunnel: w431 -> [w467 w472]
            tunnel: [w467 w471] -> w430
            tunnel: w421 -> [_ _]
            tunnel: w428 -> [_ _]
            tunnel: w425 -> [_ _]
            tunnel: w427 -> [_ _]
            tunnel: w424 -> [_ w475]
            tunnel: w422 -> [_ w476]
            tunnel: w421 -> [_ w470]
            tunnel: [w466 w469] -> w419
            tunnel: w420 -> [w466 w468]
            frame False {
            }
            frame True {
              n202 = Bundle By Name(cluster=T15 {"Point 1"={"x"=50.0, "y"=50.0}, "Point 2"={"x"=70.0, "y"=70.0}} ("Line Coordinates"), "Point 1"=w476, "Point 2"=w475) -> (w473:T15)
              n203 = call "Overlay Line with Arrows Simple.vi"("Color"=w470, "error in"=w468, "Arrows"=cluster{"Start point":bool, "End point":bool} {"Start point"=FALSE, "End point"=TRUE}, "Line Coordinates"=w473, "Image In"=w472) -> ("error out"=w469:errorcluster, "Image Out"=w471:T2)  [unwired: 5 in]
            }
          }
          n204 = call "IMAQ Overlay Line"("Color"=w421, "error in (no error)"=w419, "End Point"=w424, "Start Point"=w422, "Image"=w430) -> ("error out"=w447:errorcluster, "Image Out"=w429:T2)  [unwired: 5 in]
          n205 = call "IMAQ Convert Line to ROI"("error in (no error)"=w447, "Line"=w444) -> ("error out"=w439:errorcluster, "ROI Descriptor"=w438:T16)  [unwired: 7 in]
          n206 = call "IMAQ Edge Tool 3"("Image"=w429, "Edge Options"=w445, "Optimized Mode"=FALSE, "ROI Descriptor"=w438, "Process"=w449, "error in (no error)"=w439) -> ("Image (duplicate)"=w451:T2, "Edge Information"=w454:T18[], "Gradient Values"=w442:dbl[], "error out"=w440:errorcluster)  [unwired: 5 in, 1 out]
          n207 = call "IMAQ ROIProfile"("error in (no error)"=w440, "ROI Descriptor"=w438, "Image"=w429) -> ("error out"=w453:errorcluster, "ROI Graph"=w443:cluster{"x0":sgl, "dx":sgl, "Pixels Line":sgl[]})  [unwired: 1 in, 3 out]
          n208 = case shown="False" "單點" {
            tunnel: [w479 w490] -> w448
            tunnel: w454 -> [w481 w497]
            tunnel: [w484 w494] -> w441
            tunnel: w453 -> [w483 w492]
            tunnel: [w482 w491] -> w446
            tunnel: w451 -> [w478 w490]
            frame False {
              n209 = for {
                tunnel: w481 -> [w489] mode=indexing
                tunnel: [w488] -> w480 mode=indexing
                n210 = Unbundle By Name(w489) -> ("Location (Pixel)"=w488:cluster{"X":sgl, "Y":sgl})
              }
              n211 = Index Array(array=w481, index=0) -> (element=w485:T18)
              n212 = Unbundle By Name(w485) -> ("Location (Pixel)"=w484:cluster{"X":sgl, "Y":sgl})
              n213 = call "Overlay Points with User Specified Size.vi"("Color"=u32 16711680, "error in"=w483, "Points"=w480, "Image In"=w478) -> ("error out"=w482:errorcluster, "Image Out"=w479:T2)  [unwired: 6 in]
            }
            frame True {
              n214 = Index Array(array=w497, index=0) -> (element=w495:T18)
              n215 = Unbundle By Name(w495) -> ("Location (Pixel)"=w494:cluster{"X":sgl, "Y":sgl})
              n216 = Build Array(w494) -> (w493:cluster{"X":sgl, "Y":sgl}[])
              n217 = call "Overlay Points with User Specified Size.vi"("Color"=u32 16711680, "error in"=w492, "Points"=w493, "Image In"=w490) -> ("error out"=w491:errorcluster)  [unwired: 6 in, 1 out]
            }
          }
        }
        "Line Profile" <- w331
        n218 = flat-sequence {
          tunnel: w330 -> [w404]
          tunnel: [w404] -> w356
          tunnel: w356 -> [w406]
          frame #0 {
            n219 = property on="Gradient Information" class="WFChart (strict)"("History Data"=dbl[][] []) -> ()  [unwired: 2 in, 2 out]
          }
          frame #1 {
            n220 = Transpose 2D Array(2D array=w406) -> (transposed array=→"Gradient Information":dbl[][])
          }
        }
        n221 = for {
          tunnel: w329 -> [w410] mode=indexing
          shift-right: [w409] -> w358
          shift-left: cluster{"X":sgl, "Y":sgl}[] [] -> [w408]
          n222 = Unbundle By Name(w410) -> ("X"=w414:sgl, "Y"=w413:sgl)
          n223 = Multiply(x=w414, y=w413) -> (x*y=w412:sgl)
          n224 = Not Equal To 0?(x=w412) -> (x != 0?=w411:bool)
          n225 = case shown="True" w411 {
            tunnel: w410 -> [_ w418]
            tunnel: [w415 w417] -> w409
            tunnel: w408 -> [w415 w416]
            frame False {
            }
            frame True {
              n226 = Build Array (concatenate)(w416, w418) -> (w417:cluster{"X":sgl, "Y":sgl}[])
            }
          }
        }
        n227 = call "IMAQ Fit Line"("error in (no error)"=w327, "Pixel Radius"=sgl 10.0, "Points"=w358) -> ("error out"=w325:errorcluster, "Line Segment"=w324:T8)  [unwired: 3 in, 4 out]
        "Line Segment" <- w324
        n228 = Unbundle By Name(w324) -> ("Point 1"=w311:cluster{"X":sgl, "Y":sgl}, "Point 2"=w312:cluster{"X":sgl, "Y":sgl})
        n229 = Unbundle By Name(w311) -> ("X"=w321:sgl, "Y"=w319:sgl)
        n230 = Unbundle By Name(w312) -> ("X"=w320:sgl, "Y"=w318:sgl)
        n231 = call "IMAQ Overlay Line"("Color"=u32 16711680, "error in (no error)"=w325, "End Point"=w312, "Start Point"=w311, "Image"=w328) -> ("error out"=→"error out":errorcluster, "Image Out"=w323:T2)  [unwired: 5 in]
        n232 = Subtract(x=w318, y=w319) -> (x-y=w316:sgl)
        n233 = Subtract(x=w321, y=w320) -> (x-y=w317:sgl)
        n234 = Divide(x=w316, y=w317) -> (x/y=w315:sgl)
        n235 = Inverse Tangent(1:w315) -> (0:w314:sgl)
        n236 = expression code="(x/pi)*180.0" "radians to degrees"(w314) -> (→"degrees":sgl)
      }
    }
    "Image" <- w287
  }
